vi "Check_Size_of_Image-1.vi"(2 "error IN":errorcluster, 3 "[IN] Source Image":T1, 4 "[IN] Image for overlay":T1) -> (0 "error OUT":errorcluster, 1 "[OUT] Image for overlay":T1)   [LabVIEW 2017]
uses:
  <vilib>/vision/Image Controls.llb/IMAQ Image.ctl
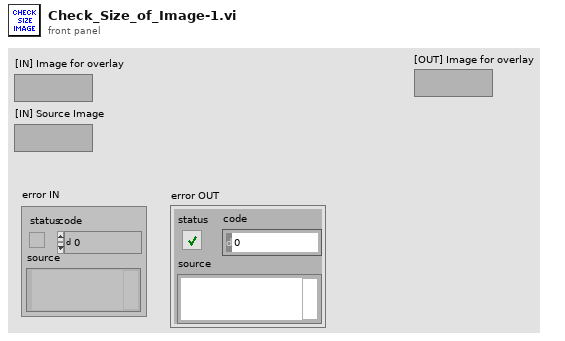
[diagram p1: front panel]
types:
  T1 = typedef "IMAQ Image.ctl" = refnum<image>
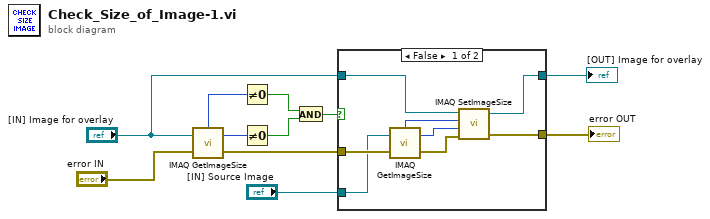
[diagram p0: block diagram]
diagram:
  n1 = call "IMAQ GetImageSize"("Image"="[IN] Image for overlay", "error in (no error)"="error IN") -> ("Y Resolution"=w10:i32, "X Resolution"=w11:i32, "error out"=w5:errorcluster)  [unwired: 2 in]
  n2 = Not Equal To 0?(x=w11) -> (x != 0?=w8:bool)
  n3 = Not Equal To 0?(x=w10) -> (x != 0?=w7:bool)
  n4 = And(x=w8, y=w7) -> (x .and. y?=w6:bool)
  n5 = case shown="False" w6 {
    tunnel: w5 -> [w17 w20]
    tunnel: "[IN] Image for overlay" -> [w15 w21]
    tunnel: [w13 w21] -> w3
    tunnel: "[IN] Source Image" -> [w14 _]
    tunnel: [w12 w20] -> w1
    frame False {
      n6 = call "IMAQ GetImageSize"("Image"=w14, "error in (no error)"=w17) -> ("Y Resolution"=w18:i32, "X Resolution"=w16:i32, "error out"=w19:errorcluster)  [unwired: 2 in]
      n7 = call "IMAQ SetImageSize"("error in (no error)"=w19, "Y Resolution"=w18, "X Resolution"=w16, "Image"=w15) -> ("error out"=w12:errorcluster, "Image Out"=w13:T1)  [unwired: 1 in]
    }
    frame True {
    }
  }
  "[OUT] Image for overlay" <- w3
  "error OUT" <- w1
